vi "principle components gp.vi"() -> ()   [LabVIEW 2013]
uses:
  <vilib>/Analysis/baseanly.llb/Real Outer Product.vi
  <vilib>/Analysis/2dsp.llb/Complex FFT.vi
  <vilib>/Analysis/2dsp.llb/Inverse Complex FFT.vi
  <vilib>/Analysis/baseanly.llb/Complex Outer Product.vi
  <vilib>/Analysis/7linalg.llb/Complex SVD Decomposition.vi
  <vilib>/Analysis/NI_AALPro.lvlib
  <vilib>/Analysis/NI_AALBase.lvlib
panel:
  out "RAW Trace":dbl[][](graph)
  out "Converted Trace":dbl[][](array[numeric])
  out "Present Err":dbl format="%#_3g"
  in  "Target Err":dbl=5e-06
  out "Itr Count":u16
  in  "Max Itr":u16=5000
  out "Spectrum":cluster{ext[], dbl[]}[](graph)
  out "Error Chart":dbl(graph)
  out "Temporal Signal":T1(graph)
  out "Recovered Trace":dbl[][](graph)
  in  "Delay Info":T2
  in  "Spectrum Info":T3
  in  "PG Test Data":dbl[][](array[numeric])=array129x256[33024 elements]
  out "Experiment Trace":dbl[][](graph)
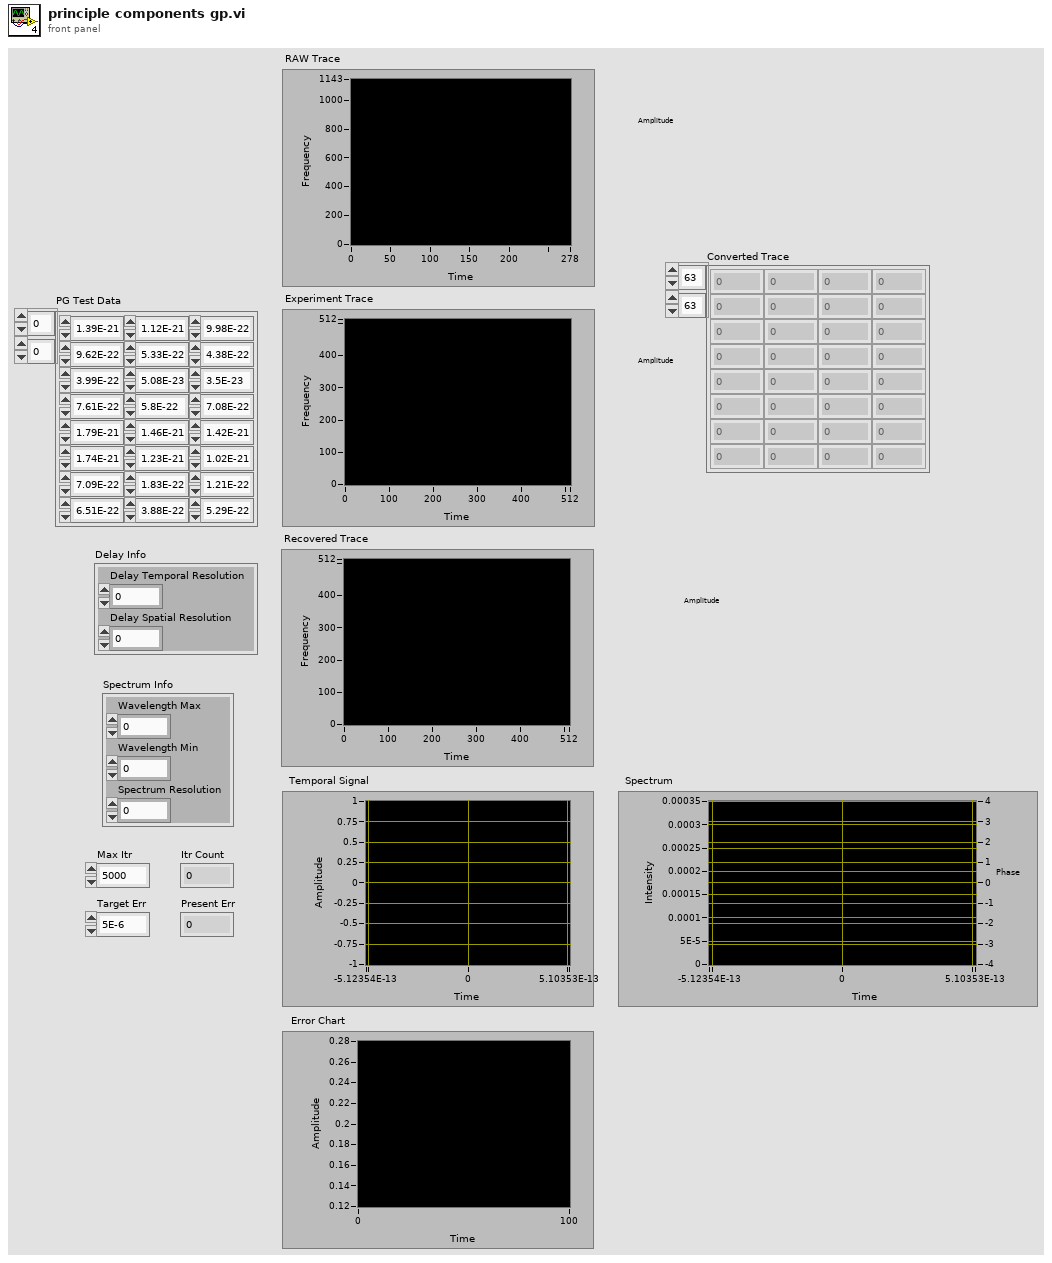
[diagram p1: front panel]
types:
  T1 = cluster{"Time Array":dbl[], "Noise Array":dbl[]}[]
  T2 = cluster{"Delay Temporal Resolution":u16, "Delay Spatial Resolution":u16}
  T3 = cluster{"Wavelength Max":dbl, "Wavelength Min":dbl, "Spectrum Resolution":u16}
  T4 = cluster{"Frequency Max":dbl, "Frequency Min":dbl, "Spectrum Resolution":u16}
  T5 = typedef "NI_Matrix.lvlib/RealMatrix.ctl" = dbl[][]
  T6 = typedef "NI_Matrix.lvlib/ComplexMatrix.ctl" = cdb[][]
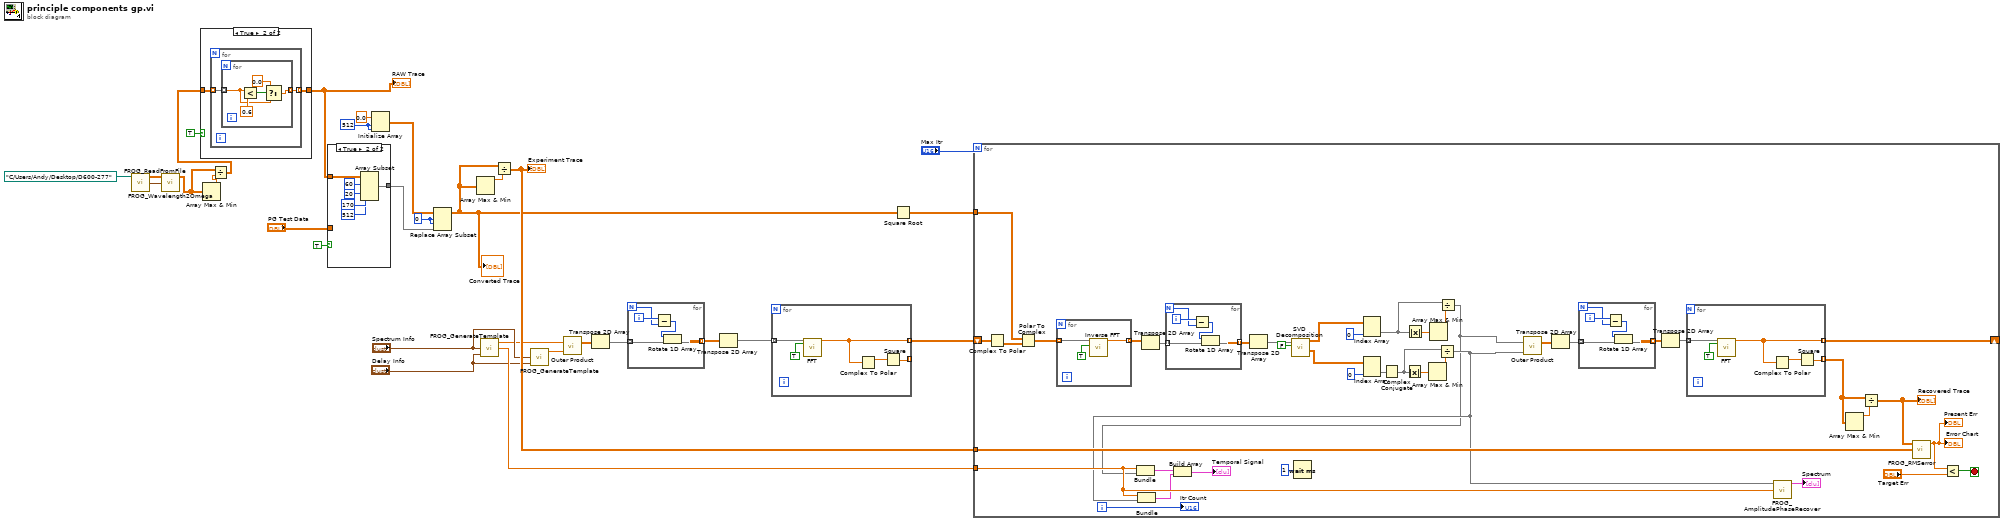
[diagram p0: block diagram]
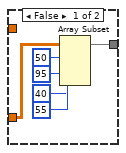
[diagram p3: hidden frame]
diagram:
  w23 = 0 ("index (row)")
  w28 = 512 ("dimension size")
  n1 = call "FROG_ReadFromFile.vi"("File Path"=path "C:/Users/Andy/Desktop/D600-277") -> ("Spectrum Info"=w6:T4, "Experiment Trace"=w4:dbl[][])  [unwired: 2 in, 1 out]
  n2 = call "FROG_Wavelength2Omega.vi"("Spectrum Info"=w6, "Experiment Trace"=w4) -> ("Converted Trace"=w2:dbl[][])  [unwired: 2 in, 1 out]
  n3 = Array Max & Min(array=w2) -> (max value=w3:dbl)  [unwired: 3 out]
  n4 = Divide(x=w2, y=w3) -> (x/y=w1:dbl[][])
  n5 = case shown="True" TRUE {
    tunnel: w1 -> [w31 w33]
    tunnel: [w31 w32] -> w8
    frame False {
    }
    frame True {
      n6 = for {
        tunnel: w33 -> [w35] mode=indexing
        tunnel: [w34] -> w32 mode=indexing
        n7 = for {
          tunnel: w35 -> [w37] mode=indexing
          tunnel: [w36] -> w34 mode=indexing
          n8 = Less?(x=w37, y=0.6) -> (x < y?=w39:bool)
          n9 = Select(t=0.0, s=w39, f=w37) -> (s? t:f=w36:dbl)
        }
      }
    }
  }
  "RAW Trace" <- w8
  n10 = case shown="True" TRUE {
    tunnel: w8 -> [_ w52]
    tunnel: [w42 w47] -> w22
    tunnel: "PG Test Data" -> [w41 _]
    frame False {
      n11 = Array Subset(array=w41, index (row)=50 ("index"), length (row)=40 ("length"), index (col)=95 ("index"), length (col)=55 ("length")) -> (w42:dbl[][])
    }
    frame True {
      n12 = Array Subset(array=w52, index (row)=60 ("index"), length (row)=170 ("length"), index (col)=20 ("index"), length (col)=512 ("length")) -> (w47:dbl[][])
    }
  }
  n13 = Initialize Array(0.0 ("element"), w28, w28) -> (w26:dbl[][])
  n14 = Replace Array Subset(array=w26, new element=w22, index (row)=w23, index (col)=w23) -> (w9:dbl[][])
  "Converted Trace" <- w9
  n15 = Array Max & Min(array=w9) -> (max value=w29:dbl)  [unwired: 3 out]
  n16 = call "FROG_GenerateTemplate.vi"("Delay Info"="Delay Info", "Spectrum Info"="Spectrum Info") -> ("Time Array"=w30:dbl[], "Noise Array"=w13:dbl[])  [unwired: 1 in, 1 out]
  n17 = Divide(x=w9, y=w29) -> (x/y=w25:dbl[][])
  "Experiment Trace" <- w25
  n18 = call "FROG_GenerateTemplate.vi"("Delay Info"="Delay Info", "Spectrum Info"="Spectrum Info") -> ("Noise Array"=w12:dbl[])  [unwired: 1 in, 2 out]
  n19 = call-poly <vilib>:"Outer Product.vi"("Y Vector"=w12, "X Vector"=w13) -> ("Outer Product"=w17:T5)  [unwired: 1 out]
  n20 = Transpose 2D Array(2D array=w17) -> (transposed array=w16:T5)
  n21 = for {
    N -> [w53]
    tunnel: w16 -> [w57] mode=indexing
    tunnel: [w56] -> w15 mode=indexing
    i -> [w54]
    n22 = Subtract(x=w54, y=w53) -> (x-y=w55:i32)
    n23 = Rotate 1D Array(1:w57, 2:w55) -> (0:w56:dbl[])
  }
  n24 = Transpose 2D Array(2D array=w15) -> (transposed array=w14:dbl[][])
  n25 = for {
    tunnel: [w58] -> w11 mode=indexing
    tunnel: w14 -> [w61] mode=indexing
    tunnel: [w59] -> _ mode=indexing
    n26 = call-poly <vilib>:"FFT.vi"("shift?"=TRUE, "X"=w61) -> ("FFT {X}"=w58:cdb[])  [unwired: 8 in, 1 out]
    n27 = Complex To Polar(r * e^(i*theta)=w58) -> (r=w60:dbl[])  [unwired: 1 out]
    n28 = Square(x=w60) -> (x^2=w59:dbl[])
  }
  n29 = Square Root(x=w9) -> (sqrt(x)=w10:dbl[][])
  n30 = for {
    N: "Max Itr" -> [_]
    tunnel: w30 -> [w97]
    tunnel: w25 -> [w87]
    tunnel: w10 -> [w76]
    shift-right: [w70] -> _
    shift-left: w11 -> [w78]
    i -> [w86]
    stop <- w83 stop-if-true
    n31 = Complex To Polar(r * e^(i*theta)=w78) -> (theta=w77:dbl[][])  [unwired: 1 out]
    n32 = Polar To Complex(1:w77, 2:w76) -> (0:w75:cdb[][])
    n33 = for {
      tunnel: w75 -> [w119] mode=indexing
      tunnel: [w121] -> w79 mode=indexing
      n34 = call-poly <vilib>:"Inverse FFT.vi"("shift?"=TRUE, "FFT {X}"=w119) -> ("X"=w121:cdb[])  [unwired: 8 in, 1 out]
    }
    n35 = Transpose 2D Array(2D array=w79) -> (transposed array=w82:cdb[][])
    n36 = for {
      N -> [w114]
      tunnel: w82 -> [w118] mode=indexing
      tunnel: [w117] -> w81 mode=indexing
      i -> [w115]
      n37 = Subtract(x=w115, y=w114) -> (x-y=w116:i32)
      n38 = Rotate 1D Array(1:w118, 2:w116) -> (0:w117:cdb[])
    }
    n39 = Transpose 2D Array(2D array=w81) -> (transposed array=w80:cdb[][])
    n40 = call-poly <vilib>:"SVD Decomposition.vi"("singular values only?"=FALSE, "A"=w80) -> ("Matrix V"=w68:T6, "Matrix U"=w67:T6)  [unwired: 5 in, 3 out]
    n41 = Wait (ms)(milliseconds to wait=u32 1) -> ()  [unwired: 1 out]
    n42 = Index Array(array=w67, index (col)=0 ("index (row)")) -> (element=w91:cdb[])  [unwired: 1 in]
    n43 = Index Array(array=w68, index (col)=0 ("index (row)")) -> (element=w100:cdb[])  [unwired: 1 in]
    n44 = Complex Conjugate(1:w100) -> (0:w88:cdb[])
    n45 = Absolute Value(x=w88) -> (abs(x)=w90:dbl[])
    n46 = Absolute Value(x=w91) -> (abs(x)=w93:dbl[])
    n47 = Array Max & Min(array=w90) -> (max value=w89:dbl)  [unwired: 3 out]
    n48 = Array Max & Min(array=w93) -> (max value=w92:dbl)  [unwired: 3 out]
    n49 = Divide(x=w88, y=w89) -> (x/y=w64:cdb[])
    n50 = Bundle("Time Array"=w97, w64) -> (w95:cluster{"Time Array":dbl[], cdb[]})  [unwired: 1 in]
    n51 = Divide(x=w91, y=w92) -> (x/y=w63:cdb[])
    n52 = Bundle("Time Array"=w97, w63) -> (w96:cluster{"Time Array":dbl[], cdb[]})  [unwired: 1 in]
    n53 = Build Array(w96, w95) -> (→"Temporal Signal":cluster{"Time Array":dbl[], cdb[]}[])
    n54 = call-poly <vilib>:"Outer Product.vi"("Y Vector"=w64, "X Vector"=w63) -> ("Outer Product"=w74:T6)  [unwired: 1 out]
    n55 = Transpose 2D Array(2D array=w74) -> (transposed array=w73:T6)
    n56 = for {
      N -> [w104]
      tunnel: w73 -> [w108] mode=indexing
      tunnel: [w107] -> w72 mode=indexing
      i -> [w105]
      n57 = Subtract(x=w105, y=w104) -> (x-y=w106:i32)
      n58 = Rotate 1D Array(1:w108, 2:w106) -> (0:w107:cdb[])
    }
    n59 = Transpose 2D Array(2D array=w72) -> (transposed array=w71:cdb[][])
    n60 = for {
      tunnel: [w109] -> w70 mode=indexing
      tunnel: w71 -> [w112] mode=indexing
      tunnel: [w110] -> w69 mode=indexing
      n61 = call-poly <vilib>:"FFT.vi"("shift?"=TRUE, "X"=w112) -> ("FFT {X}"=w109:cdb[])  [unwired: 8 in, 1 out]
      n62 = Complex To Polar(r * e^(i*theta)=w109) -> (r=w111:dbl[])  [unwired: 1 out]
      n63 = Square(x=w111) -> (x^2=w110:dbl[])
    }
    n64 = call "FROG_AmplitudePhaseRecover.vi"("Time Array"=w97, "Signal Array"=w64) -> ("Array"=→"Spectrum":cluster{ext[], dbl[]}[])  [unwired: 3 in]
    n65 = Array Max & Min(array=w69) -> (max value=w99:dbl)  [unwired: 3 out]
    n66 = Divide(x=w69, y=w99) -> (x/y=w98:dbl[][])
    "Recovered Trace" <- w98
    n67 = call "FROG_RMSerror.vi"("Experiment Trace"=w87, "Fit Trace"=w98) -> ("RMS Error"=w85:dbl)  [unwired: 1 in, 2 out]
    "Error Chart" <- w85
    "Present Err" <- w85
    n68 = Less?(x=w85, y="Target Err") -> (x < y?=w83:bool)
    "Itr Count" <- w86
  }
